vi "表面检测信息存储.vi"(8 "error in (no error)":errorcluster caption="错误输入（无错误）", 10 "OK/NG":bool, 11 "布尔":bool) -> (0 "error out":errorcluster caption="错误输出")   [LabVIEW 2017]
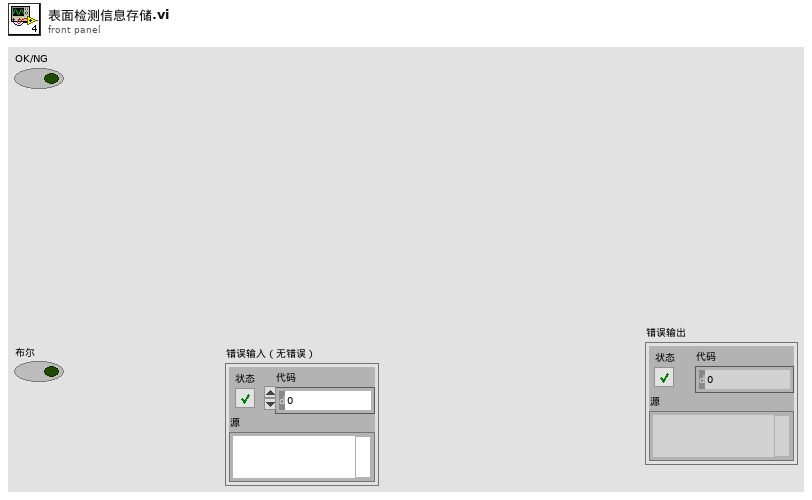
[diagram p1: front panel]
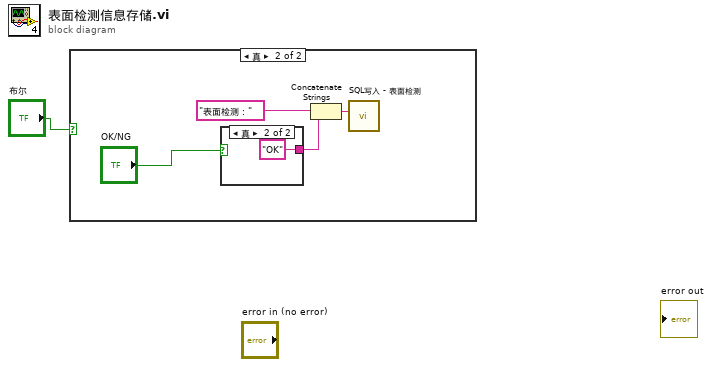
[diagram p0: block diagram]
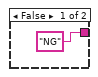
[diagram p3: hidden frame]
diagram:
  n1 = case shown="真" "布尔" {
    frame False {
    }
    frame True {
      n2 = case shown="真" "OK/NG" {
        tunnel: ["NG" "OK"] -> w3
        frame False {
        }
        frame True {
        }
      }
      n3 = Concatenate Strings("表面检测：", w3) -> (w4:string)
      n4 = call "SQL写入 - 表面检测.vi"("TestMessage"=w4) -> ()  [unwired: 14 in, 1 out]
    }
  }
